vi "Power Off Positions.vi"(8 "error in (no error)":errorcluster, 10 "Power Off All":bool, 11 "Driver Test":refnum<class "Driver Test.lvclass">) -> (0 "error out":errorcluster)   [LabVIEW 2015, in "Driver Test.lvclass"]
doc: "Opens switch route to all non-running positions."
uses:
  Driver Test.lvclass
  Classes/Application/Class/Application.lvclass
  Test Class/Test Class.lvclass
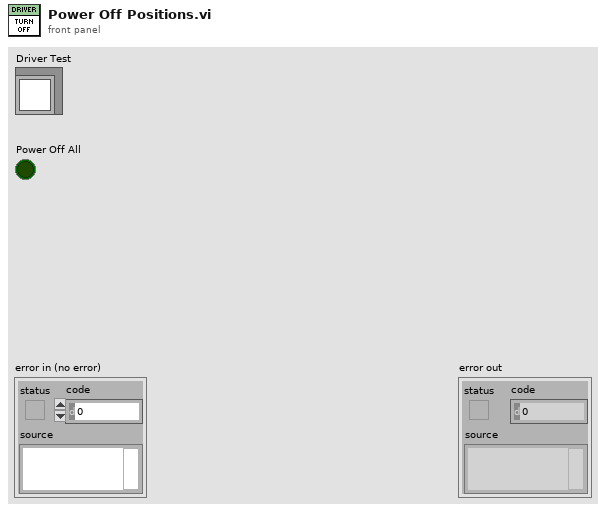
[diagram p1: front panel]
types:
  T1 = cluster{"Serial Number Reference":refnum<vi>, "Status Message Reference":refnum<vi>, "Position":u32}[]
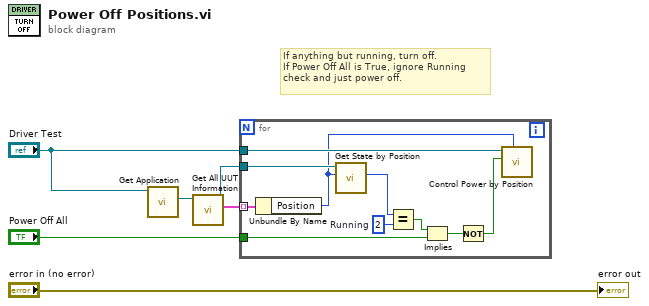
[diagram p0: block diagram]
diagram:
  # "If anything but running, turn off.\nIf Power Off All is True, ignore Running\ncheck and just power off."
  n1 = call "Get Application.vi"("Test Class in"="Driver Test") -> ("Application.lvlib:Application.lvclass"=w2:refnum<class "Application.lvclass">)  [unwired: 9 in, 1 out]
  n2 = call-dynamic "Get All UUT Information.vi"("Application in"=w2) -> ("All UUTs"=w5:T1, "Application out"=w3:refnum<class "Application.lvclass">)  [unwired: 8 in, 1 out]
  n3 = for {
    tunnel: w5 -> [w16] mode=indexing
    tunnel: w3 -> [w15]
    tunnel: "Power Off All" -> [w12]
    tunnel: "Driver Test" -> [w9]
    w14 = u32 2  # Running
    n4 = Unbundle By Name(w16) -> ("Position"=w8:u32)
    n5 = call-dynamic "Get State by Position.vi"("Position"=w8, "Application in"=w15) -> ("State"=w10:u32)  [unwired: 7 in, 2 out]
    n6 = Equal?(x=w10, y=w14) -> (x = y?=w13:bool)
    n7 = Implies(1:w12, 2:w13) -> (0:w11:bool)
    n8 = Not(x=w11) -> (.not. x?=w7:bool)
    n9 = call "Control Power by Position.vi"("Position"=w8, "Power On?"=w7, "Driver Test in"=w9) -> ()  [unwired: 8 in, 1 out]
  }
  "error out" <- "error in (no error)"
